vi "Hide.vi"(8 "error in (no error)":errorcluster, 11 "SMO.UI_Embed In":refnum<class "SMO.UI_Embed.lvclass">) -> (0 "error out":errorcluster, 3 "SMO.UI_Embed Out":refnum<class "SMO.UI_Embed.lvclass">)   [LabVIEW 2019, in "SMO.UI_Embed.lvclass"]
doc: "Closes the front panel of the SMO.UI_Embed or removes it from the subpanel (based on how it was open).\nNote that this method does not stop the Process.vi."
uses:
  SMO.UI_Embed.lvclass
  Typedefs/SMO.UI_Embed State--enum.ctl
panel:
  # "For instructions on how to use the JKI State Machine Objects, examples and video tutorials, visit:\nhttp://jki.net/state-machine-objects/\n\nJKI State Machine Objects™\nhttp://jki.net/state-machine-objects/\nCopyright (C) 2005-2015, JKI <info@jki.net>\nALL RIGHTS RESERVED"
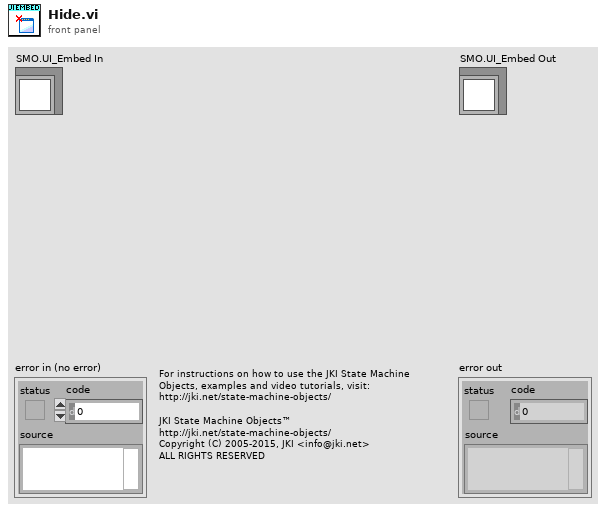
[diagram p1: front panel]
types:
  T1 = typedef "SMO.UI_Embed.lvclass/SMO.UI_Embed State--enum.ctl" = enum16{"unknown", "Opened", "Embedded", "Closed"}
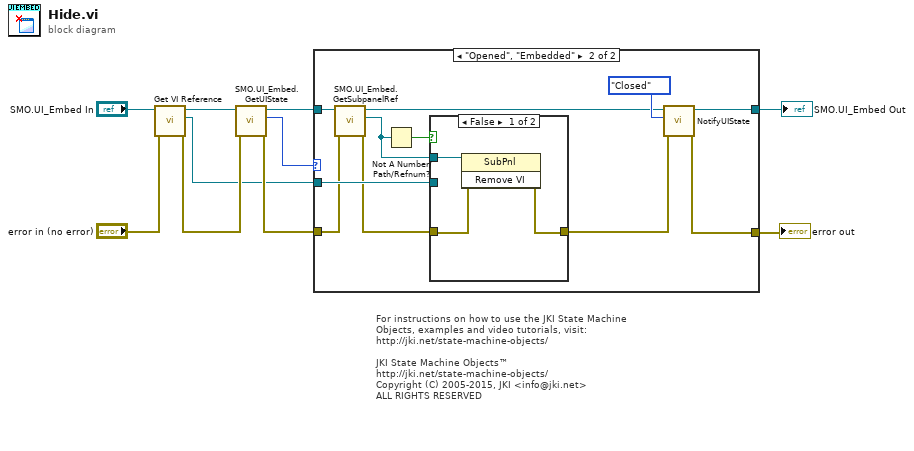
[diagram p0: block diagram]
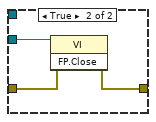
[diagram p3: hidden frame]
diagram:
  # "For instructions on how to use the JKI State Machine Objects, examples and video tutorials, visit:\nhttp://jki.net/state-machine-objects/\n\nJKI State Machine Objects™\nhttp://jki.net/state-machine-objects/\nCopyright (C) 2005-2015, JKI <info@jki.net>\nALL RIGHTS RESERVED"
  n1 = call-dynamic "Get VI Reference.vi"("error in (no error)"="error in (no error)", "SMO.UI_Embed In"="SMO.UI_Embed In") -> ("error out"=w2:errorcluster, "VI Reference"=w1:refnum<vi>, "SMO.UI_Embed Out"=w4:refnum<class "SMO.UI_Embed.lvclass">)  [unwired: 7 in]
  n2 = call "SMO.UI_Embed.GetUIState.vi"("error in (no error)"=w2, "SMO.UI_Embed In"=w4) -> ("error out"=w6:errorcluster, "UI State"=w7:T1, "SMO.UI_Embed Out"=w8:refnum<class "SMO.UI_Embed.lvclass">)  [unwired: 7 in]
  n3 = case shown="\"Opened\", \"Embedded\"" w7 {
    tunnel: [w11 w13] -> w10
    tunnel: [w12 w14] -> w9
    tunnel: w8 -> [w12 w22]
    tunnel: w1 -> [_ w18]
    tunnel: w6 -> [w11 w16]
    frame Default {
    }
    frame "Opened", "Embedded" {
      n4 = call "SMO.UI_Embed.GetSubpanelRef.vi"("error in (no error)"=w16, "SMO.UI_Embed In"=w22) -> ("error out"=w15:errorcluster, "Subpanel Ref"=w17:refnum<vi>, "SMO.UI_Embed Out"=w21:refnum<class "SMO.UI_Embed.lvclass">)  [unwired: 7 in]
      n5 = Not A Number/Path/Refnum?(number/path/refnum=w17) -> (NaN/Path/Refnum?=w19:bool)
      n6 = case shown="False" w19 {
        tunnel: w15 -> [w26 w28]
        tunnel: [w25 w27] -> w20
        tunnel: w18 -> [_ w29]
        tunnel: w17 -> [w24 _]
        frame False {
          n7 = invoke class="SubPnl" method="Remove VI"(reference=w24, error in=w26) -> (error out=w25:errorcluster)  [unwired: 1 in, 2 out]
        }
        frame True {
          n8 = invoke class="VI" method="FP.Close"(reference=w29, error in=w28) -> (error out=w27:errorcluster)  [unwired: 1 in, 2 out]
        }
      }
      n9 = call "NotifyUIState.vi"("error in (no error)"=w20, "UI State"=SMO.UI_Embed_State--enum."Closed", "SMO.UI_Embed In"=w21) -> ("error out"=w13:errorcluster, "SMO.UI_Embed Out"=w14:refnum<class "SMO.UI_Embed.lvclass">)  [unwired: 7 in]
    }
  }
  "error out" <- w10
  "SMO.UI_Embed Out" <- w9
